vi "Msg to Send.vi"(10 "Events":T1) -> (3 "Panel Event Msg out":refnum<class "Panel Event Msg.lvclass">)   [LabVIEW 2021, in "Panel Event.lvlib" / "Panel Event Msg.lvclass"]
uses:
  Panel Event Msg.lvclass
  Events.ctl
  Panel Event Msg.lvclass/Panel Event Msg.ctl
  Panel Event.lvlib
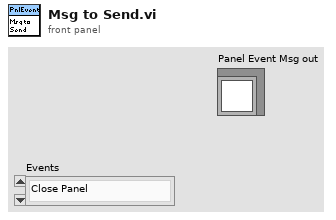
[diagram p1: front panel]
types:
  T1 = typedef "Panel Event.lvlib/Events.ctl" = enum16{"Close Panel", "Show Panel", "Hide Panel"}
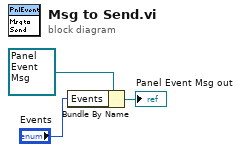
[diagram p0: block diagram]
diagram:
  n1 = Bundle By Name(cluster=refnum<class "Panel Event Msg.lvclass"> refnum ("Panel Event Msg in"), "Events"="Events") -> (→"Panel Event Msg out":refnum<class "Panel Event Msg.lvclass">)
